vi "modbus_module.vi"(8 "error in (no error)":errorcluster, 10 "User Event":T1, 11 "queue in":T2) -> (0 "error out":errorcluster)   [LabVIEW 2019]
uses:
  core_dataRef.ctl
  core_dataCluster.ctl
  gui/modbus_data_notifier.ctl
  instrument/instr_dataCluster.ctl
  instrument/Instrument.lvclass
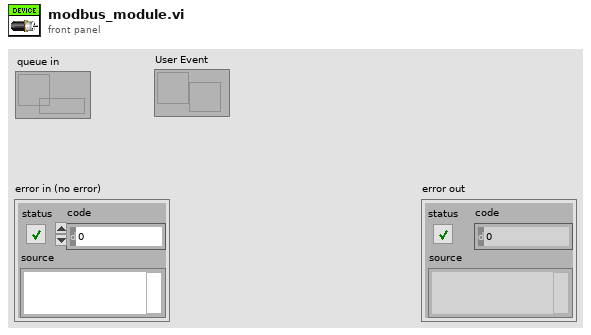
[diagram p1: front panel]
types:
  T1 = typedef "modbus_data_notifier.ctl" = refnum<notifier>
  T2 = typedef "core_dataRef.ctl" = refnum<queue>
  T3 = cluster{"voltage":sgl, "current":sgl, "ovp":sgl, "ocp":sgl, "Enable":bool}
  T4 = typedef "core_dataCluster.ctl" = cluster{"cmd":string, "data":variant}
  T5 = typedef "Instrument.lvclass/instr_dataCluster.ctl" = cluster{"电源电压 V":dbl, "电源电流A":dbl, "扭矩N/m":dbl, "速度r/M":dbl, "温度℃":dbl[], "流量计L/M":dbl[]}
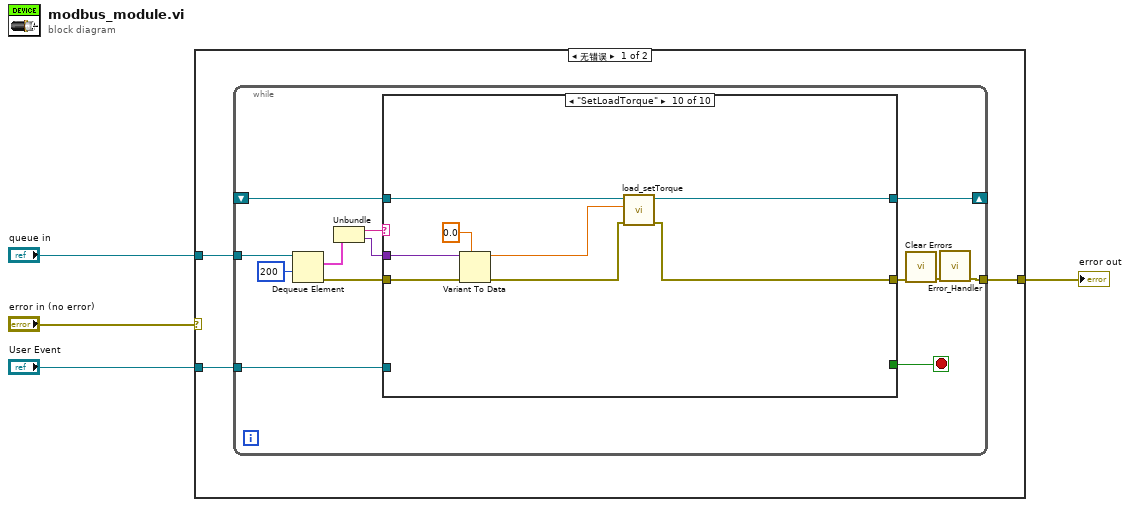
[diagram p0: block diagram]
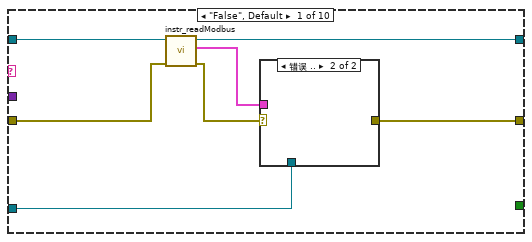
[diagram p2: hidden frame]
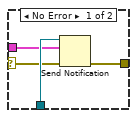
[diagram p3: hidden frame]
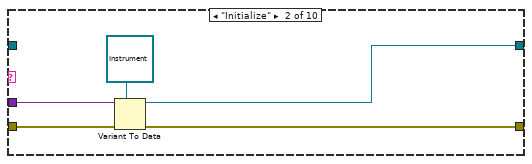
[diagram p4: hidden frame]
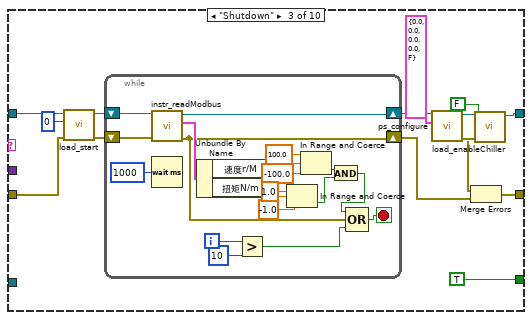
[diagram p5: hidden frame]
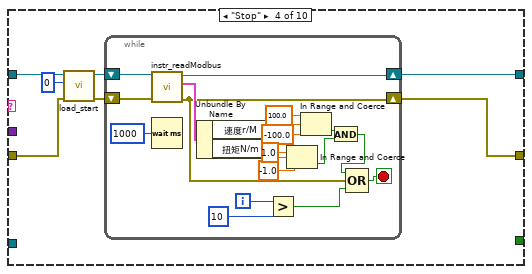
[diagram p6: hidden frame]
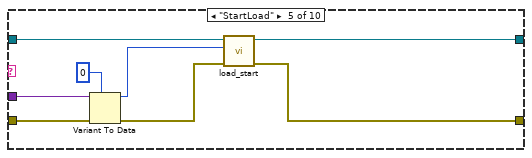
[diagram p7: hidden frame]
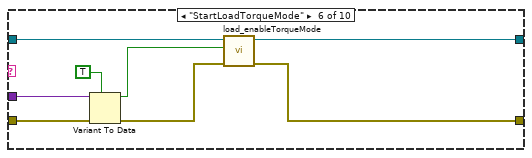
[diagram p8: hidden frame]
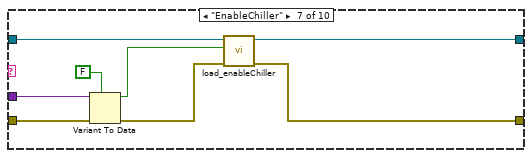
[diagram p9: hidden frame]
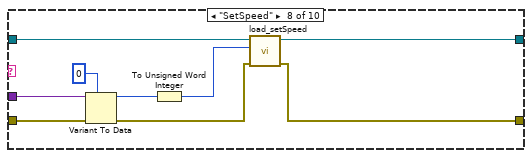
[diagram p10: hidden frame]
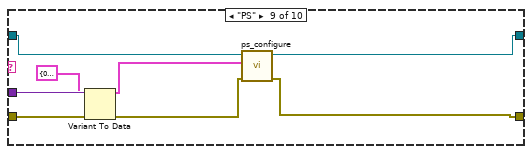
[diagram p11: hidden frame]
diagram:
  n1 = case shown="无错误" "error in (no error)" {
    selector: "error in (no error)" -> [_ w146]
    tunnel: "queue in" -> [w7 _]
    tunnel: [w6 w146] -> w3
    tunnel: "User Event" -> [w5 _]
    frame No Error {
      n2 = while {
        tunnel: w7 -> [w20]
        shift-right: [w15] -> _
        shift-left: _ -> [w14]
        tunnel: [w11] -> w6
        tunnel: w5 -> [w9]
        stop <- w13 stop-if-true
        n3 = Dequeue Element(queue=w20, timeout in ms (-1)=200) -> (element=w19:T4, error out=w17:errorcluster)  [unwired: 1 in, 2 out]
        n4 = Unbundle(w19) -> ("cmd"=w18:string, "data"=w16:variant)
        n5 = case shown="\"SetLoadTorque\"" w18 {
          tunnel: w17 -> [w25 w36 w49 w76 w101 w109 w117 w129 w135 w145]
          tunnel: w16 -> [_ w35 _ _ w99 w107 w115 w128 w132 w144]
          tunnel: [w26 w33 w37 w72 w103 w111 w119 w123 w136 w140] -> w15
          tunnel: w14 -> [w27 _ w50 w77 w104 w112 w120 w126 w137 w142]
          tunnel: [w24 w32 w44 w71 w102 w110 w118 w122 w133 w139] -> w12
          tunnel: [_ _ TRUE _ _ _ _ _ _ _] -> w13
          tunnel: w9 -> [w23 _ _ _ _ _ _ _ _ _]
          frame "False", Default {
            n6 = call "instr_readModbus.vi"("error in (no error)"=w25, "Instrument in"=w27) -> ("error out"=w21:errorcluster, "Cluster"=w22:T5, "Instrument out"=w26:refnum<class "Instrument.lvclass">)  [unwired: 7 in]
            n7 = case shown="错误 .." w21 {
              selector: w21 -> [w28 _]
              tunnel: [w31 _] -> w24
              tunnel: w23 -> [w30 _]
              tunnel: w22 -> [w29 _]
              frame No Error {
                n8 = Send Notification(notification=w29, notifier=w30, error in (no error)=w28) -> (error out=w31:errorcluster)  [unwired: 1 out]
              }
              frame Error {
              }
            }
          }
          frame "Initialize" {
            n9 = Variant To Data(error in=w36, type=refnum<class "Instrument.lvclass"> refnum ("Instrument.lvclass"), Variant=w35) -> (data=w33:refnum<class "Instrument.lvclass">, error out=w32:errorcluster)
          }
          frame "Shutdown" {
            n10 = call "load_start.vi"("error in (no error)"=w49, "start"=i16 0, "Instrument in"=w50) -> ("error out"=w46:errorcluster, "Instrument out"=w47:refnum<class "Instrument.lvclass">)  [unwired: 7 in]
            n11 = while {
              shift-right: [w67] -> w45
              shift-left: w47 -> [w70]
              shift-right: [w66] -> w43
              shift-left: w46 -> [w69]
              i -> [w54]
              stop <- w65 stop-if-true
              n12 = call "instr_readModbus.vi"("error in (no error)"=w69, "Instrument in"=w70) -> ("error out"=w66:errorcluster, "Cluster"=w68:T5, "Instrument out"=w67:refnum<class "Instrument.lvclass">)  [unwired: 7 in]
              n13 = Wait (ms)(milliseconds to wait=u32 1000) -> ()  [unwired: 1 out]
              n14 = Unbundle By Name(w68) -> ("速度r/M"=w64:dbl, "扭矩N/m"=w63:dbl)
              n15 = Greater?(x=w54, y=10) -> (0:w52:bool)
              n16 = In Range and Coerce(upper limit=1.0, x=w63, lower limit=-1.0) -> (In Range?=w61:bool)  [unwired: 1 out]
              n17 = In Range and Coerce(upper limit=100.0, x=w64, lower limit=-100.0) -> (In Range?=w62:bool)  [unwired: 1 out]
              n18 = And(x=w62, y=w61) -> (x .and. y?=w60:bool)
              n19 = Compound Arithmetic op=OR(w60, w66, w52) -> (w65:bool)
            }
            n20 = call "ps_configure.vi"("SET PS"=T3 {"voltage"=0.0, "current"=0.0, "ovp"=0.0, "ocp"=0.0, "Enable"=FALSE}, "Instrument in"=w45) -> ("error out"=w41:errorcluster, "Instrument out"=w40:refnum<class "Instrument.lvclass">)  [unwired: 8 in]
            n21 = call "load_enableChiller.vi"("error in (no error)"=w41, "start"=FALSE, "Instrument in"=w40) -> ("error out"=w39:errorcluster, "Instrument out"=w37:refnum<class "Instrument.lvclass">)  [unwired: 7 in]
            n22 = Merge Errors(w39, w43) -> (w44:errorcluster)
          }
          frame "Stop" {
            n23 = call "load_start.vi"("error in (no error)"=w76, "start"=i16 0, "Instrument in"=w77) -> ("error out"=w73:errorcluster, "Instrument out"=w74:refnum<class "Instrument.lvclass">)  [unwired: 7 in]
            n24 = while {
              shift-right: [w93] -> w72
              shift-left: w74 -> [w96]
              shift-right: [w92] -> w71
              shift-left: w73 -> [w95]
              i -> [w80]
              stop <- w91 stop-if-true
              n25 = call "instr_readModbus.vi"("error in (no error)"=w95, "Instrument in"=w96) -> ("error out"=w92:errorcluster, "Cluster"=w94:T5, "Instrument out"=w93:refnum<class "Instrument.lvclass">)  [unwired: 7 in]
              n26 = Wait (ms)(milliseconds to wait=u32 1000) -> ()  [unwired: 1 out]
              n27 = Unbundle By Name(w94) -> ("速度r/M"=w90:dbl, "扭矩N/m"=w89:dbl)
              n28 = Greater?(x=w80, y=10) -> (0:w78:bool)
              n29 = In Range and Coerce(upper limit=1.0, x=w89, lower limit=-1.0) -> (In Range?=w87:bool)  [unwired: 1 out]
              n30 = In Range and Coerce(upper limit=100.0, x=w90, lower limit=-100.0) -> (In Range?=w88:bool)  [unwired: 1 out]
              n31 = And(x=w88, y=w87) -> (x .and. y?=w86:bool)
              n32 = Compound Arithmetic op=OR(w86, w92, w78) -> (w91:bool)
            }
          }
          frame "StartLoad" {
            n33 = Variant To Data(error in=w101, type=i16 0, Variant=w99) -> (data=w97:i16, error out=w100:errorcluster)
            n34 = call "load_start.vi"("error in (no error)"=w100, "start"=w97, "Instrument in"=w104) -> ("error out"=w102:errorcluster, "Instrument out"=w103:refnum<class "Instrument.lvclass">)  [unwired: 7 in]
          }
          frame "StartLoadTorqueMode" {
            n35 = Variant To Data(error in=w109, type=TRUE, Variant=w107) -> (data=w105:bool, error out=w108:errorcluster)
            n36 = call "load_enableTorqueMode.vi"("error in (no error)"=w108, "enable"=w105, "Instrument in"=w112) -> ("error out"=w110:errorcluster, "Instrument out"=w111:refnum<class "Instrument.lvclass">)  [unwired: 7 in]
          }
          frame "EnableChiller" {
            n37 = Variant To Data(error in=w117, type=FALSE, Variant=w115) -> (data=w113:bool, error out=w116:errorcluster)
            n38 = call "load_enableChiller.vi"("error in (no error)"=w116, "start"=w113, "Instrument in"=w120) -> ("error out"=w118:errorcluster, "Instrument out"=w119:refnum<class "Instrument.lvclass">)  [unwired: 7 in]
          }
          frame "SetSpeed" {
            n39 = Variant To Data(error in=w129, type=0, Variant=w128) -> (data=w125:i32, error out=w124:errorcluster)
            n40 = To Unsigned Word Integer(number=w125) -> (unsigned 16bit integer=w121:u16)
            n41 = call "load_setSpeed.vi"("error in (no error)"=w124, "loadSpeed"=w121, "Instrument in"=w126) -> ("error out"=w122:errorcluster, "Instrument out"=w123:refnum<class "Instrument.lvclass">)  [unwired: 7 in]
          }
          frame "PS" {
            n42 = Variant To Data(error in=w135, type=T3 {"voltage"=0.0, "current"=0.0, "ovp"=0.0, "ocp"=0.0, "Enable"=FALSE} ("类型"), Variant=w132) -> (data=w131:T3, error out=w134:errorcluster)
            n43 = call "ps_configure.vi"("error in (no error)"=w134, "SET PS"=w131, "Instrument in"=w137) -> ("error out"=w133:errorcluster, "Instrument out"=w136:refnum<class "Instrument.lvclass">)  [unwired: 7 in]
          }
          frame "SetLoadTorque" {
            n44 = Variant To Data(error in=w145, type=0.0, Variant=w144) -> (data=w138:dbl, error out=w141:errorcluster)
            n45 = call "load_setTorque.vi"("error in (no error)"=w141, "torque set"=w138, "Instrument in"=w142) -> ("error out"=w139:errorcluster, "Instrument out"=w140:refnum<class "Instrument.lvclass">)  [unwired: 7 in]
          }
        }
        n46 = call <vilib>:"Clear Errors.vi"("error in (no error)"=w12) -> ("error out"=w8:errorcluster)  [unwired: 5 in, 1 out]
        n47 = call "Error_Handler.vi"("error in"=w8) -> ("error out"=w11:errorcluster)  [unwired: 8 in, 2 out]
      }
    }
    frame Error {
    }
  }
  "error out" <- w3
